vi "Add Object.vi"(8 "error in (no error)":errorcluster, 9 "Datatype":T1, 10 "Name":string, 11 "Objects in":refnum<class "Objects.lvclass">) -> (0 "error out":errorcluster, 3 "Objects out":refnum<class "Objects.lvclass">)   [LabVIEW 2019, in "HierDAL Library.lvlib" / "Database.lvlib" / "Repositories.lvlib" / "Objects.lvclass"]
uses:
  Objects.lvclass
  Common Library/Controls/Datatype.ctl
  Objects.lvclass/Objects.ctl
  Database Manager Class/Database Manager.lvclass
  Common Library/Common.lvlib
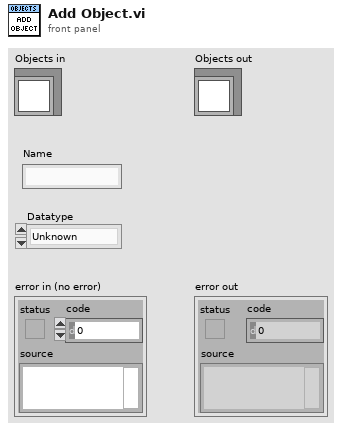
[diagram p1: front panel]
types:
  T1 = typedef "HierDAL Library.lvlib/Common.lvlib/Datatype.ctl" = enum16{"Unknown", "Group", "Dataset"}
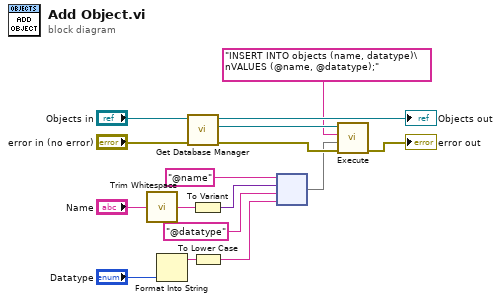
[diagram p0: block diagram]
diagram:
  n1 = call <vilib>:"Trim Whitespace.vi"("string"="Name") -> ("trimmed string"=w1:string)  [unwired: 1 in]
  n2 = Format Into String("Datatype") -> (resulting string=w12:string)  [unwired: 3 in, 1 out]
  n3 = call "Get Database Manager.vi"("error in (no error)"="error in (no error)", "Objects in"="Objects in") -> ("error out"=w5:errorcluster, "Database Manager"=w4:refnum<class "Database Manager.lvclass">, "Objects out"=→"Objects out":refnum<class "Objects.lvclass">)  [unwired: 7 in]
  n4 = To Variant(anything=w1) -> (Variant=w11:variant)
  n5 = To Lower Case(string=w12) -> (all lower case string=w7:string)
  n6 = node("@name" ("key"), w11, "@datatype" ("key"), w7) -> (w2:map{string, variant})
  n7 = call-dynamic "Execute.vi"("error in (no error)"=w5, "Parameters"=w2, "Query"="INSERT INTO objects (name, datatype)\nVALUES (@name, @datatype);", "Database Manager in"=w4) -> ("error out"=→"error out":errorcluster)  [unwired: 6 in, 1 out]
